vi "plot_init.vi"(10 "簇":T1, 11 "配置输入":T2 {"串口通信UI"."Format" items=["标准帧", "扩展帧"]; "串口通信UI"."Type" items=["数据帧", "远程帧"]; "串口通信UI"."ID" format="0x%x"; "串口通信UI"."Fliter" items=["接收所有类型"=1, "只接收标准帧"=2, "只接收扩展帧"=3]; "串口通信UI"."kBaudRate" items=["5k bps"=1, "10k bps"=2, "20k bps"=3, "40k bps"=4, "50k bps"=5, "80k bps"=6, "100k bps"=7, "125k bps"=8, "200k bps"=9, "250k bps"=10, "400k bps"=11, "500k bps"=12, "666k bps"=13, "800k bps"=14, "1000k bps"=15, "33.33k bps"=16, "66.66k bps"=17, "83.33k bps"=18]; "串口通信UI"."Mode" items=["正常工作", "仅侦听模式", "自测模式（环回）"]; "串口通信UI"."InitFlag" items=["使用界面设置参数"=1]; "串口通信UI"."AccMask" format="%08x"; "串口通信UI"."AccCode" format="%08x"; "串口通信UI"."Channel" items=["通道1", "通道2"]; "串口通信UI"."DevType" items=["USB-CAN"=3, "USB-CAN2"=4]; "安全报警UI"."操作 8" items=["产生报警信息（不发声），等待手动操作", "产生报警信息（发声），等待手动操作", "产生报警信息（不发声），自动刹车", "产生报警信息（发声），自动刹车", "产生报警信息（不发声），立即自动断电，开启泄放电阻", "产生报警信息（发声），立即自动断电，开启泄放电阻"]; "安全报警UI"."操作 7" items=["产生报警信息（不发声），等待手动操作", "产生报警信息（发声），等待手动操作", "产生报警信息（不发声），自动刹车", "产生报警信息（发声），自动刹车", "产生报警信息（不发声），立即自动断电，开启泄放电阻", "产生报警信息（发声），立即自动断电，开启泄放电阻"]; "安全报警UI"."操作 6" items=["产生报警信息（不发声），等待手动操作", "产生报警信息（发声），等待手动操作", "产生报警信息（不发声），自动刹车", "产生报警信息（发声），自动刹车", "产生报警信息（不发声），立即自动断电，开启泄放电阻", "产生报警信息（发声），立即自动断电，开启泄放电阻"]; "安全报警UI"."操作 5" items=["产生报警信息（不发声），等待手动操作", "产生报警信息（发声），等待手动操作", "产生报警信息（不发声），自动刹车", "产生报警信息（发声），自动刹车", "产生报警信息（不发声），立即自动断电，开启泄放电阻", "产生报警信息（发声），立即自动断电，开启泄放电阻"]; "安全报警UI"."操作 4" items=["产生报警信息（不发声），等待手动操作", "产生报警信息（发声），等待手动操作", "产生报警信息（不发声），自动刹车", "产生报警信息（发声），自动刹车", "产生报警信息（不发声），立即自动断电，开启泄放电阻", "产生报警信息（发声），立即自动断电，开启泄放电阻"]; "安全报警UI"."操作 3" items=["产生报警信息（不发声），等待手动操作", "产生报警信息（发声），等待手动操作", "产生报警信息（不发声），自动刹车", "产生报警信息（发声），自动刹车", "产生报警信息（不发声），立即自动断电，开启泄放电阻", "产生报警信息（发声），立即自动断电，开启泄放电阻"]; "安全报警UI"."操作 2" items=["产生报警信息（不发声），等待手动操作", "产生报警信息（发声），等待手动操作", "产生报警信息（不发声），自动刹车", "产生报警信息（发声），自动刹车", "产生报警信息（不发声），立即自动断电，开启泄放电阻", "产生报警信息（发声），立即自动断电，开启泄放电阻"]; "安全报警UI"."操作" items=["产生报警信息（不发声），等待手动操作", "产生报警信息（发声），等待手动操作", "产生报警信息（不发声），自动刹车", "产生报警信息（发声），自动刹车", "产生报警信息（不发声），立即自动断电，开启泄放电阻", "产生报警信息（发声），立即自动断电，开启泄放电阻"]}) -> (3 "配置输出":T2 {"串口通信UI"."Format" items=["标准帧", "扩展帧"]; "串口通信UI"."Type" items=["数据帧", "远程帧"]; "串口通信UI"."ID" format="0x%x"; "串口通信UI"."Fliter" items=["接收所有类型"=1, "只接收标准帧"=2, "只接收扩展帧"=3]; "串口通信UI"."kBaudRate" items=["5k bps"=1, "10k bps"=2, "20k bps"=3, "40k bps"=4, "50k bps"=5, "80k bps"=6, "100k bps"=7, "125k bps"=8, "200k bps"=9, "250k bps"=10, "400k bps"=11, "500k bps"=12, "666k bps"=13, "800k bps"=14, "1000k bps"=15, "33.33k bps"=16, "66.66k bps"=17, "83.33k bps"=18]; "串口通信UI"."Mode" items=["正常工作", "仅侦听模式", "自测模式（环回）"]; "串口通信UI"."InitFlag" items=["使用界面设置参数"=1]; "串口通信UI"."AccMask" format="%08x"; "串口通信UI"."AccCode" format="%08x"; "串口通信UI"."Channel" items=["通道1", "通道2"]; "串口通信UI"."DevType" items=["USB-CAN"=3, "USB-CAN2"=4]; "安全报警UI"."操作 8" items=["产生报警信息（不发声），等待手动操作", "产生报警信息（发声），等待手动操作", "产生报警信息（不发声），自动刹车", "产生报警信息（发声），自动刹车", "产生报警信息（不发声），立即自动断电，开启泄放电阻", "产生报警信息（发声），立即自动断电，开启泄放电阻"]; "安全报警UI"."操作 7" items=["产生报警信息（不发声），等待手动操作", "产生报警信息（发声），等待手动操作", "产生报警信息（不发声），自动刹车", "产生报警信息（发声），自动刹车", "产生报警信息（不发声），立即自动断电，开启泄放电阻", "产生报警信息（发声），立即自动断电，开启泄放电阻"]; "安全报警UI"."操作 6" items=["产生报警信息（不发声），等待手动操作", "产生报警信息（发声），等待手动操作", "产生报警信息（不发声），自动刹车", "产生报警信息（发声），自动刹车", "产生报警信息（不发声），立即自动断电，开启泄放电阻", "产生报警信息（发声），立即自动断电，开启泄放电阻"]; "安全报警UI"."操作 5" items=["产生报警信息（不发声），等待手动操作", "产生报警信息（发声），等待手动操作", "产生报警信息（不发声），自动刹车", "产生报警信息（发声），自动刹车", "产生报警信息（不发声），立即自动断电，开启泄放电阻", "产生报警信息（发声），立即自动断电，开启泄放电阻"]; "安全报警UI"."操作 4" items=["产生报警信息（不发声），等待手动操作", "产生报警信息（发声），等待手动操作", "产生报警信息（不发声），自动刹车", "产生报警信息（发声），自动刹车", "产生报警信息（不发声），立即自动断电，开启泄放电阻", "产生报警信息（发声），立即自动断电，开启泄放电阻"]; "安全报警UI"."操作 3" items=["产生报警信息（不发声），等待手动操作", "产生报警信息（发声），等待手动操作", "产生报警信息（不发声），自动刹车", "产生报警信息（发声），自动刹车", "产生报警信息（不发声），立即自动断电，开启泄放电阻", "产生报警信息（发声），立即自动断电，开启泄放电阻"]; "安全报警UI"."操作 2" items=["产生报警信息（不发声），等待手动操作", "产生报警信息（发声），等待手动操作", "产生报警信息（不发声），自动刹车", "产生报警信息（发声），自动刹车", "产生报警信息（不发声），立即自动断电，开启泄放电阻", "产生报警信息（发声），立即自动断电，开启泄放电阻"]; "安全报警UI"."操作" items=["产生报警信息（不发声），等待手动操作", "产生报警信息（发声），等待手动操作", "产生报警信息（不发声），自动刹车", "产生报警信息（发声），自动刹车", "产生报警信息（不发声），立即自动断电，开启泄放电阻", "产生报警信息（发声），立即自动断电，开启泄放电阻"]})   [LabVIEW 2018, in "UI.lvlib"]
uses:
  UI.lvlib
  Settings/Settings.ctl
  Acquisition/Hardware Configuration.ctl
  Acquisition/Signal Type.ctl
  Acquisition/Acquisition.lvlib
  Settings/Settings.lvlib
panel:
  # "参数配置文件"
  # "输入数据文件"
  # "EHA电机"
  # "模拟电机"
  # "注：每次运行实验时销毁现有所有图像"
  # "参数配置文件"
  # "输入数据文件"
  # "EHA电机"
  # "模拟电机"
  # "注：每次运行实验时销毁现有所有图像"
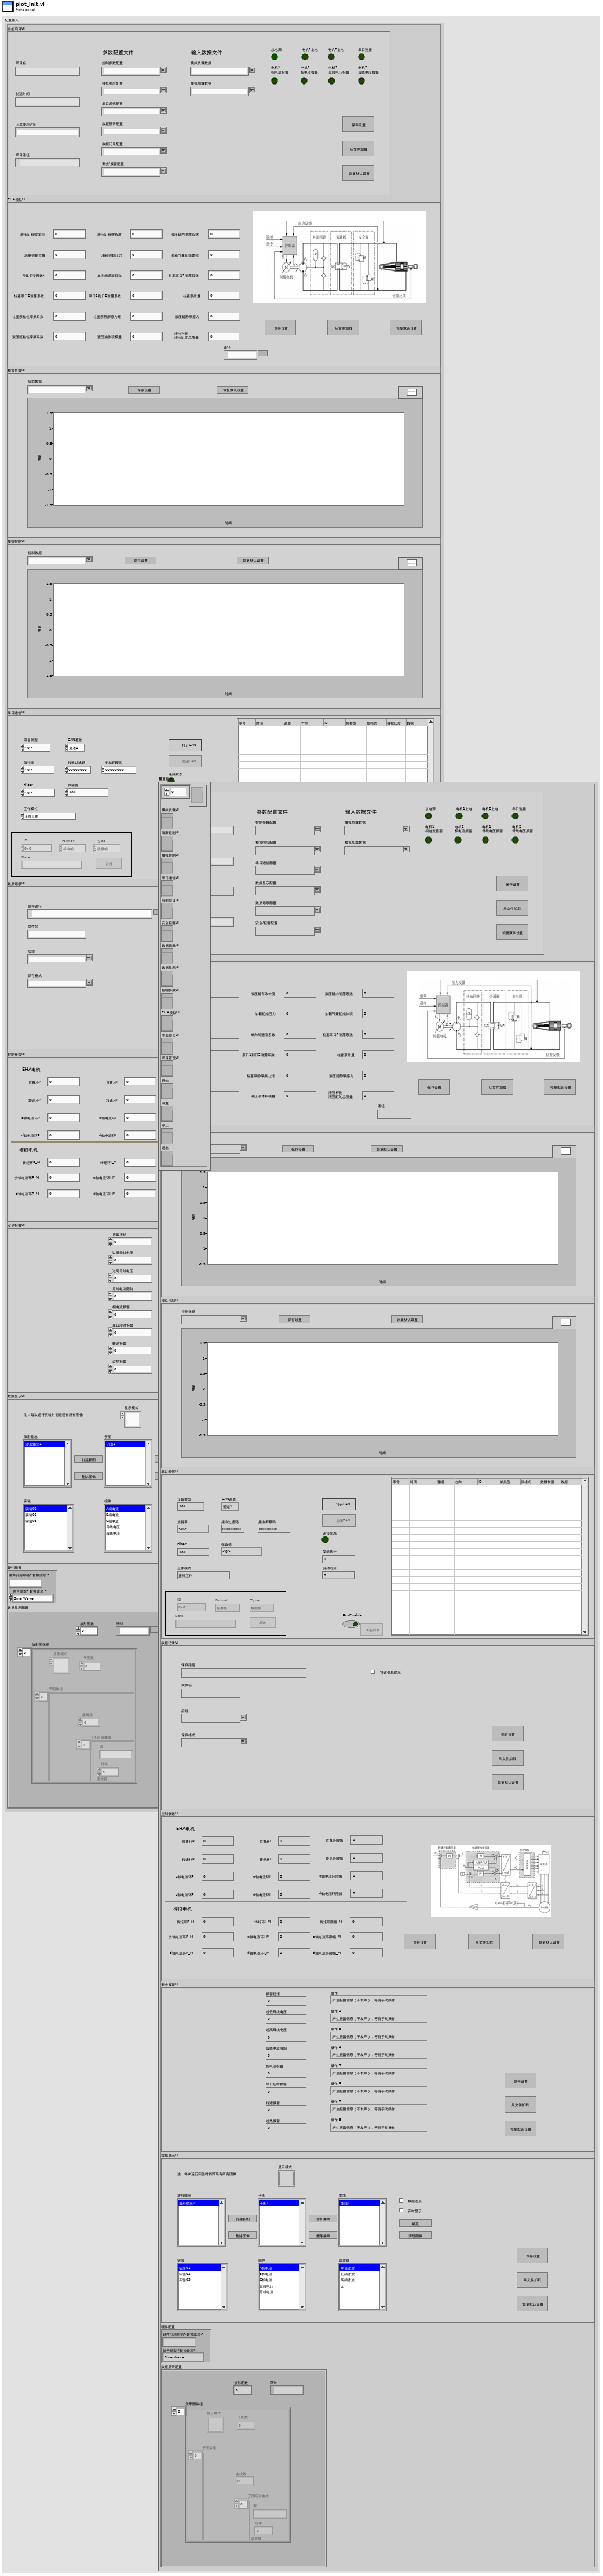
[diagram p1: front panel]
types:
  T1 = typedef "引用簇.ctl" = cluster{"数组":refnum<vi>[], "模拟负载UI":refnum<vi>, "波形控制UI":refnum<vi>, "模拟控制UI":refnum<vi>, "串口通信UI":refnum<vi>, "当前项目UI":refnum<vi>, "安全报警UI":refnum<vi>, "数据记录UI":refnum<vi>, "数据显示UI":refnum<vi>, "控制参数UI":refnum<vi>, "EHA模拟UI":refnum<vi>, "主选项卡UI":refnum<vi>, "项目管理UI":refnum<vi>, "开始":refnum<vi>, "设置":refnum<vi>, "停止":refnum<vi>, "退出":refnum<vi>}
  T2 = typedef "Settings.lvlib/Settings.ctl" = cluster{"当前项目UI":T3, "EHA模拟UI":T4, "模拟负载UI":T5, "模拟控制UI":T6, "串口通信UI":T7, "数据记录UI":T13, "控制参数UI":T14, "安全报警UI":T15, "数据显示UI":T16, "硬件配置":T17, "数据显示配置":T19}
  T3 = typedef "控件 5.ctl" = cluster{"控制参数配置":string, "模拟响应配置":string, "串口通信配置":string, "数据显示配置":string, "数据记录配置":string, "安全/报警配置":string, "模拟负载数据":string, "模拟加载数据":string, "总电源":bool, "电机1上电":bool, "电机2上电":bool, "串口连接":bool, "电机1\n相电流报警":bool, "电机2\n相电流报警":bool, "电机1\n母线电压报警":bool, "电机2\n母线电压报警":bool, "保存设置":bool, "从文件加载":bool, "恢复默认设置":bool, "路径":path, "项目路径":path, "项目名":string, "创建时间":string, "上次使用时间":string}
  T4 = typedef "EHA模拟UI.ctl" = cluster{"液压缸有效面积":dbl, "活塞初始位置":dbl, "气体多变系数k":dbl, "柱塞泵口2泄露系数":dbl, "柱塞泵粘性摩擦系数":dbl, "液压缸粘性摩擦系数":dbl, "液压缸有效长度":dbl, "油箱初始压力":dbl, "单向阀通流系数":dbl, "泵口1到口2泄露系数":dbl, "柱塞泵静摩擦力矩":dbl, "液压油体积模量":dbl, "保存设置":bool, "从文件加载":bool, "恢复默认设置":bool, "路径":path, "液压缸内泄露系数":dbl, "油箱气囊初始体积":dbl, "柱塞泵口1泄露系数":dbl, "柱塞泵排量":dbl, "液压缸静摩擦力":dbl, "液压杆到\n液压缸的总质量":dbl}
  T5 = typedef "控件 9.ctl" = cluster{"负载数据":string, "负载数据 2":waveform(dbl)[], "保存设置":bool, "恢复默认设置":bool}
  T6 = typedef "控件 7.ctl" = cluster{"控制数据":string, "负载数据 2":waveform(dbl)[], "保存设置":bool, "恢复默认设置":bool}
  T7 = typedef "控件 6.ctl" = cluster{"DevType":T8, "Channel":T9, "AccCode":u32, "AccMask":u32, "InitFlag":T10, "Mode":T11, "kBaudRate":u8, "Fliter":T12, "Open":bool, "Close":bool, "连接状态":bool, "SendCnt":u32, "RecvCnt":u32, "Send":bool, "ID":u32, "Data":string, "Type":u8, "Format":u8, "Clear":bool, "list":i32, "路径":path, "RcvEnable":bool}
  T8 = typedef "can库.lvlib/ControlCAN.lvlib/DevType.ctl" = u32
  T9 = typedef "can库.lvlib/ControlCAN.lvlib/CAN Channel.ctl" = u32
  T10 = typedef "can库.lvlib/ControlCAN.lvlib/InitFlag.ctl" = u32
  T11 = typedef "can库.lvlib/ControlCAN.lvlib/Mode.ctl" = u8
  T12 = typedef "can库.lvlib/ControlCAN.lvlib/Fliter.ctl" = u8
  T13 = typedef "控件 3.ctl" = cluster{"保存路径":path, "文件名":string, "后缀":string, "保存格式":string, "复选框":bool, "保存设置":bool, "从文件加载":bool, "恢复默认设置":bool, "路径":path, "TDMS文件引用":refnum<k34>}
  T14 = typedef "控件 1.ctl" = cluster{"d轴电流环P_M":dbl, "转速环P":dbl, "q轴电流环P":dbl, "d轴电流环P":dbl, "转矩环P_M":dbl, "去轴电流环P_M":dbl, "转速环I":dbl, "q轴电流环I":dbl, "d轴电流环I":dbl, "转矩环I_M":dbl, "q轴电流环I_M":dbl, "d轴电流环I_M":dbl, "保存设置":bool, "从文件加载":bool, "恢复默认设置":bool, "路径":path, "位置环P":dbl, "位置环I":dbl, "转速环限幅":dbl, "q轴电流环限幅":dbl, "d轴电流环限幅":dbl, "位置环限幅":dbl, "转矩环限幅_M":dbl, "q轴电流环限幅_M":dbl, "d轴电流环限幅_M":dbl}
  T15 = typedef "控件 4.ctl" = cluster{"报警扭矩":dbl, "过低母线电压":dbl, "过高母线电压":dbl, "母线电流限制":dbl, "相电流报警":dbl, "串口超时报警":dbl, "转速报警":dbl, "过热报警":dbl, "操作":u16, "操作 2":u16, "操作 3":u16, "操作 4":u16, "操作 5":u16, "操作 6":u16, "操作 7":u16, "操作 8":u16, "保存设置":bool, "从文件加载":bool, "恢复默认设置":bool, "路径":path}
  T16 = typedef "控件 2.ctl" = cluster{"保存设置":bool, "从文件加载":bool, "恢复默认设置":bool, "实验":i32, "波形输出":i32, "组件":i32, "曲线":i32, "滤波器":i32, "删除曲线":bool, "清理图像":bool, "添加曲线":bool, "数据选点":bool, "确定按钮":bool, "实时显示":bool, "子图":i32, "显示模式":u16, "路径":path, "删除图像":bool, "创建新图":bool}
  T17 = typedef "Acquisition.lvlib/Hardware Configuration.ctl" = cluster{"硬件引用句柄<替换此项>":string, "信号类型<替换该项>":T18}
  T18 = typedef "Acquisition.lvlib/Signal Type.ctl" = enum16{"Sine Wave", "Square with Noise"}
  T19 = typedef "波形图簇.ctl" = cluster{"波形图数":u32, "波形图数组":T20[], "路径":path}
  T20 = typedef "波形图.ctl" = cluster{"显示模式":u16, "子图数":u32, "子图数组":T21[]}
  T21 = typedef "子图.ctl" = cluster{"子图所有曲线":T22[], "曲线数":u32}
  T22 = typedef "曲线簇.ctl" = cluster{"源":string, "组件":u32, "滤波器":u32}
  T23 = typedef "主选项卡枚举常量.ctl" = enum32{"开始页", "当前项目配置", "串口通信配置", "控制参数配置", "EHA模拟配置", "模拟控制配置", "模拟负载配置", "安全报警配置", "数据显示配置", "数据记录配置", "波形输出1", "波形输出2", "波形输出3", "波形输出4", "波形输出5", "波形输出6"}
  T24 = typedef "组件常量.ctl" = string[]
  T25 = enum32{"开始页", "当前项目配置", "串口通信配置", "控制参数配置", "模拟响应配置", "模拟控制配置", "模拟负载配置", "安全报警配置", "数据显示配置", "数据记录配置", "波形输出1", "波形输出2", "波形输出3", "波形输出4", "波形输出5", "波形输出6"}
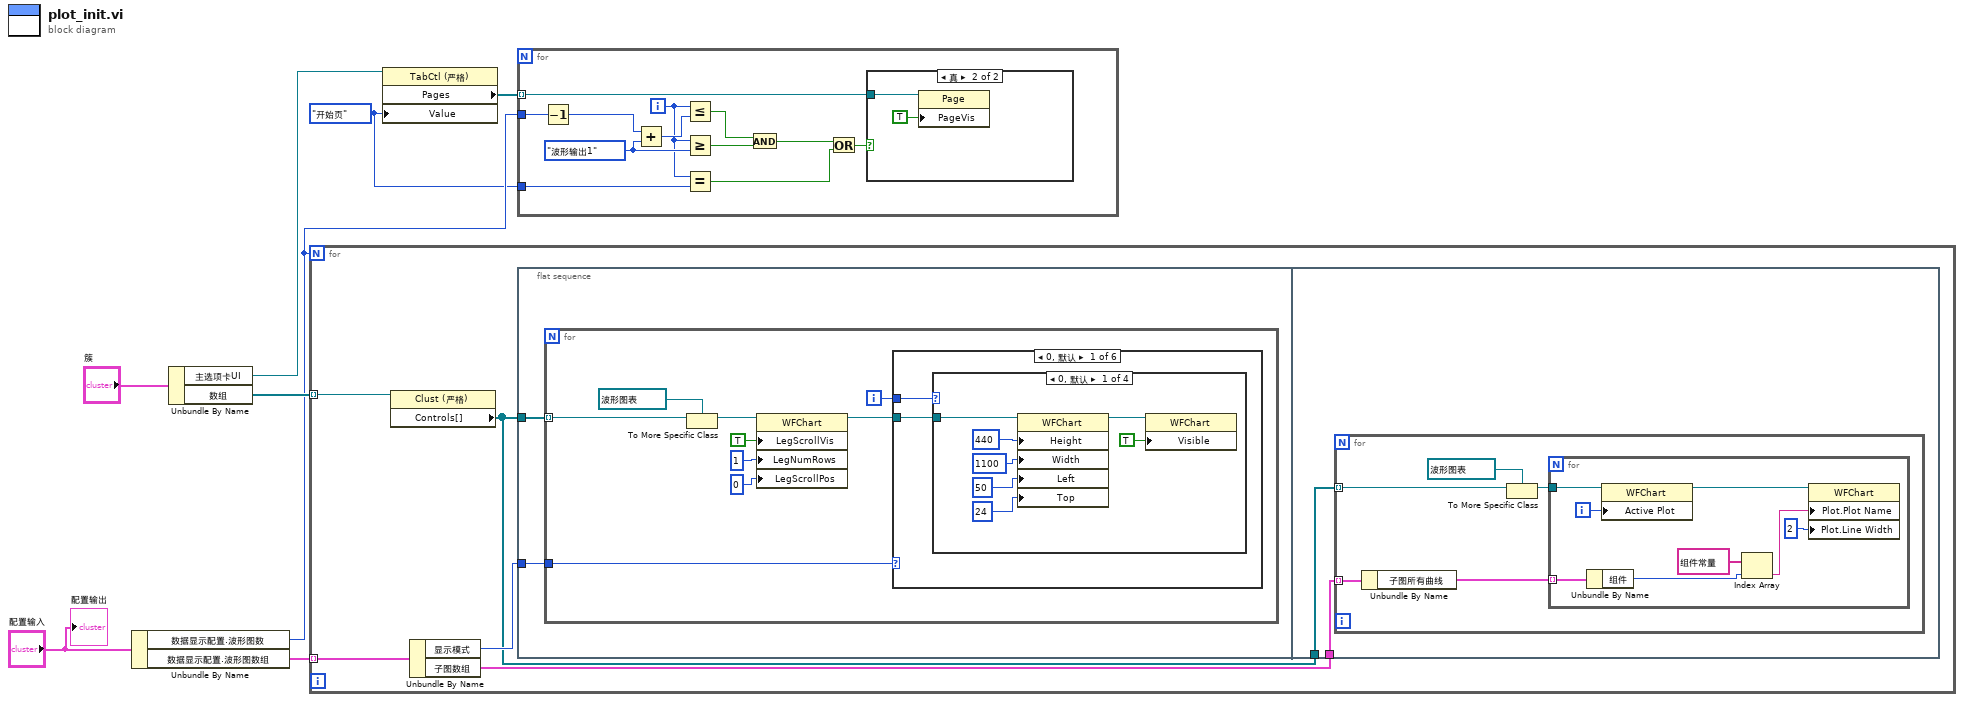
[diagram p0: block diagram]
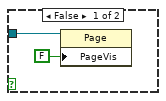
[diagram p2: hidden frame]
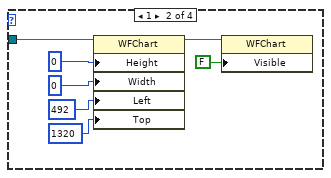
[diagram p3: hidden frame]
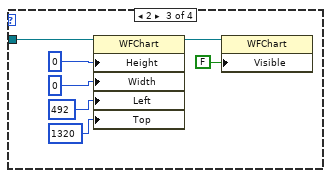
[diagram p4: hidden frame]
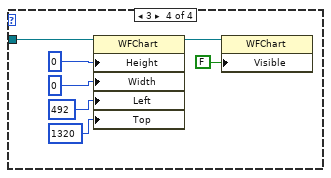
[diagram p5: hidden frame]
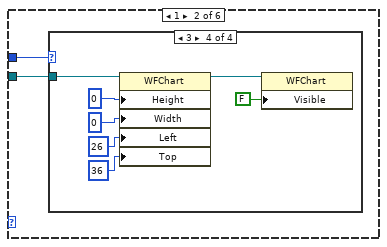
[diagram p6: hidden frame]
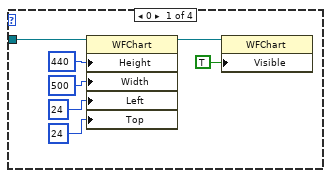
[diagram p7: hidden frame]
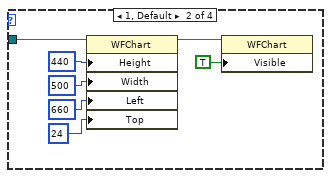
[diagram p8: hidden frame]
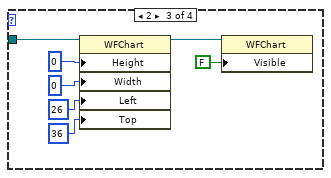
[diagram p9: hidden frame]
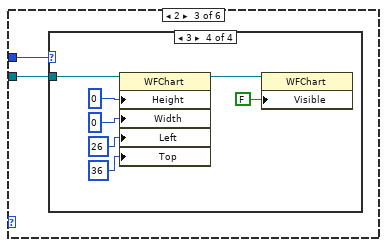
[diagram p10: hidden frame]
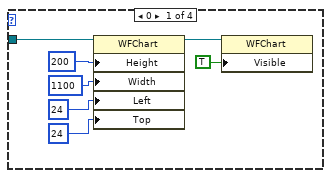
[diagram p11: hidden frame]
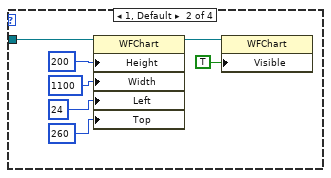
[diagram p12: hidden frame]
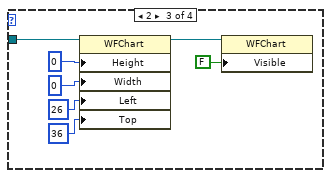
[diagram p13: hidden frame]
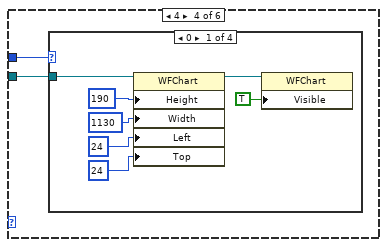
[diagram p14: hidden frame]
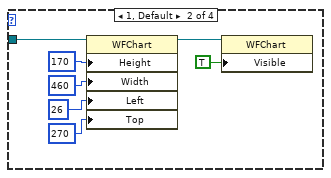
[diagram p15: hidden frame]
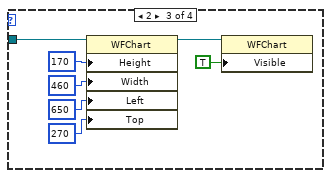
[diagram p16: hidden frame]
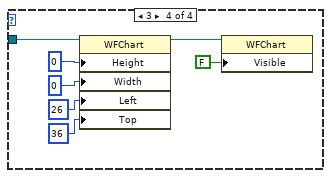
[diagram p17: hidden frame]
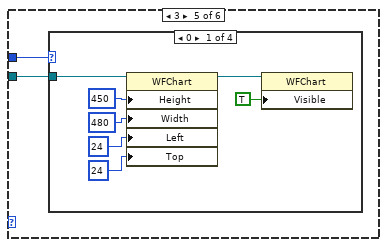
[diagram p18: hidden frame]
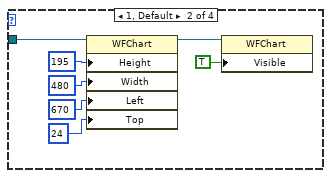
[diagram p19: hidden frame]
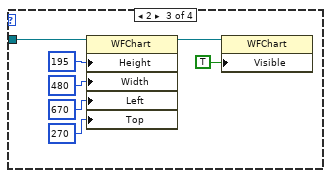
[diagram p20: hidden frame]
diagram:
  w1 = 主选项卡枚举常量."开始页" ("值")
  n1 = Unbundle By Name("配置输入") -> ("数据显示配置.波形图数"=w2:u32, "数据显示配置.波形图数组"=w6:T20[])
  n2 = Unbundle By Name("簇") -> ("主选项卡UI"=w4:refnum<vi>, "数组"=w5:refnum<vi>[])
  n3 = for {
    N: w2 -> [_]
    tunnel: w6 -> [w13] mode=indexing
    tunnel: w5 -> [w11] mode=indexing
    n4 = property class="Clust (严格)"(reference=w11) -> ("Controls[]"=w9:refnum<vi>[])  [unwired: 1 in, 2 out]
    n5 = Unbundle By Name(w13) -> ("显示模式"=w12:u16, "子图数组"=w10:T21[])
    n6 = flat-sequence {
      tunnel: w12 -> [w15]
      tunnel: w9 -> [w14]
      tunnel: w10 -> [w206]
      tunnel: w9 -> [w205]
      frame #0 {
        n7 = for {
          tunnel: w15 -> [w20]
          tunnel: w14 -> [w16] mode=indexing
          i -> [w19]
          n8 = To More Specific Class(target class=refnum<vi> refnum ("特定类引用"), reference=w16) -> (specific class reference=w18:refnum<vi>)  [unwired: 1 in, 1 out]
          n9 = property class="WFChart"(reference=w18, "LegScrollVis"=TRUE ("图例:滚动条可见"), "LegNumRows"=u32 1 ("图例:行数"), "LegScrollPos"=u32 0 ("图例:滚动条位置")) -> (reference out=w17:refnum<vi>)  [unwired: 1 in, 1 out]
          n10 = case shown="0, 默认" w20 {
            tunnel: w19 -> [w26 w56 w86 w116 w146 w176]
            tunnel: w17 -> [w25 w55 w85 w115 w145 w175]
            frame 0, Default {
              n11 = case shown="0, 默认" w26 {
                tunnel: w25 -> [w29 w34 w41 w48]
                frame 0, Default {
                  n12 = property class="WFChart"(reference=w29, "Height"=u32 440 ("绘图区域:大小:高度"), "Width"=u32 1100 ("绘图区域:大小:宽度"), "Left"=50 ("位置:居左"), "Top"=24 ("x")) -> (reference out=w27:refnum<vi>)  [unwired: 1 in, 1 out]
                  n13 = property class="WFChart"(reference=w27, "Visible"=TRUE ("可见")) -> ()  [unwired: 1 in, 2 out]
                }
                frame 1 {
                  n14 = property class="WFChart"(reference=w34, "Height"=u32 0 ("绘图区域:大小:高度"), "Width"=u32 0 ("绘图区域:大小:宽度"), "Left"=492 ("位置:居左"), "Top"=1320 ("x")) -> (reference out=w35:refnum<vi>)  [unwired: 1 in, 1 out]
                  n15 = property class="WFChart"(reference=w35, "Visible"=FALSE ("可见")) -> ()  [unwired: 1 in, 2 out]
                }
                frame 2 {
                  n16 = property class="WFChart"(reference=w41, "Height"=u32 0 ("绘图区域:大小:高度"), "Width"=u32 0 ("绘图区域:大小:宽度"), "Left"=492 ("位置:居左"), "Top"=1320 ("x")) -> (reference out=w42:refnum<vi>)  [unwired: 1 in, 1 out]
                  n17 = property class="WFChart"(reference=w42, "Visible"=FALSE ("可见")) -> ()  [unwired: 1 in, 2 out]
                }
                frame 3 {
                  n18 = property class="WFChart"(reference=w48, "Height"=u32 0 ("绘图区域:大小:高度"), "Width"=u32 0 ("绘图区域:大小:宽度"), "Left"=492 ("位置:居左"), "Top"=1320 ("x")) -> (reference out=w49:refnum<vi>)  [unwired: 1 in, 1 out]
                  n19 = property class="WFChart"(reference=w49, "Visible"=FALSE ("可见")) -> ()  [unwired: 1 in, 2 out]
                }
              }
            }
            frame 1 {
              n20 = case shown="3" w56 {
                tunnel: w55 -> [w57 w64 w71 w78]
                frame 0 {
                  n21 = property class="WFChart"(reference=w57, "Height"=u32 440 ("绘图区域:大小:高度"), "Width"=u32 500 ("绘图区域:大小:宽度"), "Left"=24 ("位置:居左"), "Top"=24 ("x")) -> (reference out=w58:refnum<vi>)  [unwired: 1 in, 1 out]
                  n22 = property class="WFChart"(reference=w58, "Visible"=TRUE ("可见")) -> ()  [unwired: 1 in, 2 out]
                }
                frame 1, Default {
                  n23 = property class="WFChart"(reference=w64, "Height"=u32 440 ("绘图区域:大小:高度"), "Width"=u32 500 ("绘图区域:大小:宽度"), "Left"=660 ("位置:居左"), "Top"=24 ("x")) -> (reference out=w65:refnum<vi>)  [unwired: 1 in, 1 out]
                  n24 = property class="WFChart"(reference=w65, "Visible"=TRUE ("可见")) -> ()  [unwired: 1 in, 2 out]
                }
                frame 2 {
                  n25 = property class="WFChart"(reference=w71, "Height"=u32 0 ("绘图区域:大小:高度"), "Width"=u32 0 ("绘图区域:大小:宽度"), "Left"=26 ("位置:居左"), "Top"=36 ("x")) -> (reference out=w72:refnum<vi>)  [unwired: 1 in, 1 out]
                  n26 = property class="WFChart"(reference=w72, "Visible"=FALSE ("可见")) -> ()  [unwired: 1 in, 2 out]
                }
                frame 3 {
                  n27 = property class="WFChart"(reference=w78, "Height"=u32 0 ("绘图区域:大小:高度"), "Width"=u32 0 ("绘图区域:大小:宽度"), "Left"=26 ("位置:居左"), "Top"=36 ("x")) -> (reference out=w79:refnum<vi>)  [unwired: 1 in, 1 out]
                  n28 = property class="WFChart"(reference=w79, "Visible"=FALSE ("可见")) -> ()  [unwired: 1 in, 2 out]
                }
              }
            }
            frame 2 {
              n29 = case shown="3" w86 {
                tunnel: w85 -> [w87 w94 w101 w108]
                frame 0 {
                  n30 = property class="WFChart"(reference=w87, "Height"=u32 200 ("绘图区域:大小:高度"), "Width"=u32 1100 ("绘图区域:大小:宽度"), "Left"=24 ("位置:居左"), "Top"=24 ("x")) -> (reference out=w88:refnum<vi>)  [unwired: 1 in, 1 out]
                  n31 = property class="WFChart"(reference=w88, "Visible"=TRUE ("可见")) -> ()  [unwired: 1 in, 2 out]
                }
                frame 1, Default {
                  n32 = property class="WFChart"(reference=w94, "Height"=u32 200 ("绘图区域:大小:高度"), "Width"=u32 1100 ("绘图区域:大小:宽度"), "Left"=24 ("位置:居左"), "Top"=260 ("x")) -> (reference out=w95:refnum<vi>)  [unwired: 1 in, 1 out]
                  n33 = property class="WFChart"(reference=w95, "Visible"=TRUE ("可见")) -> ()  [unwired: 1 in, 2 out]
                }
                frame 2 {
                  n34 = property class="WFChart"(reference=w101, "Height"=u32 0 ("绘图区域:大小:高度"), "Width"=u32 0 ("绘图区域:大小:宽度"), "Left"=26 ("位置:居左"), "Top"=36 ("x")) -> (reference out=w102:refnum<vi>)  [unwired: 1 in, 1 out]
                  n35 = property class="WFChart"(reference=w102, "Visible"=FALSE ("可见")) -> ()  [unwired: 1 in, 2 out]
                }
                frame 3 {
                  n36 = property class="WFChart"(reference=w108, "Height"=u32 0 ("绘图区域:大小:高度"), "Width"=u32 0 ("绘图区域:大小:宽度"), "Left"=26 ("位置:居左"), "Top"=36 ("x")) -> (reference out=w109:refnum<vi>)  [unwired: 1 in, 1 out]
                  n37 = property class="WFChart"(reference=w109, "Visible"=FALSE ("可见")) -> ()  [unwired: 1 in, 2 out]
                }
              }
            }
            frame 4 {
              n38 = case shown="0" w116 {
                tunnel: w115 -> [w117 w124 w131 w138]
                frame 0 {
                  n39 = property class="WFChart"(reference=w117, "Height"=u32 190 ("绘图区域:大小:高度"), "Width"=u32 1130 ("绘图区域:大小:宽度"), "Left"=24 ("位置:居左"), "Top"=24 ("x")) -> (reference out=w118:refnum<vi>)  [unwired: 1 in, 1 out]
                  n40 = property class="WFChart"(reference=w118, "Visible"=TRUE ("可见")) -> ()  [unwired: 1 in, 2 out]
                }
                frame 1, Default {
                  n41 = property class="WFChart"(reference=w124, "Height"=u32 170 ("绘图区域:大小:高度"), "Width"=u32 460 ("绘图区域:大小:宽度"), "Left"=26 ("位置:居左"), "Top"=270 ("x")) -> (reference out=w125:refnum<vi>)  [unwired: 1 in, 1 out]
                  n42 = property class="WFChart"(reference=w125, "Visible"=TRUE ("可见")) -> ()  [unwired: 1 in, 2 out]
                }
                frame 2 {
                  n43 = property class="WFChart"(reference=w131, "Height"=u32 170 ("绘图区域:大小:高度"), "Width"=u32 460 ("绘图区域:大小:宽度"), "Left"=650 ("位置:居左"), "Top"=270 ("x")) -> (reference out=w132:refnum<vi>)  [unwired: 1 in, 1 out]
                  n44 = property class="WFChart"(reference=w132, "Visible"=TRUE ("可见")) -> ()  [unwired: 1 in, 2 out]
                }
                frame 3 {
                  n45 = property class="WFChart"(reference=w138, "Height"=u32 0 ("绘图区域:大小:高度"), "Width"=u32 0 ("绘图区域:大小:宽度"), "Left"=26 ("位置:居左"), "Top"=36 ("x")) -> (reference out=w139:refnum<vi>)  [unwired: 1 in, 1 out]
                  n46 = property class="WFChart"(reference=w139, "Visible"=FALSE ("可见")) -> ()  [unwired: 1 in, 2 out]
                }
              }
            }
            frame 3 {
              n47 = case shown="0" w146 {
                tunnel: w145 -> [w147 w154 w161 w168]
                frame 0 {
                  n48 = property class="WFChart"(reference=w147, "Height"=u32 450 ("绘图区域:大小:高度"), "Width"=u32 480 ("绘图区域:大小:宽度"), "Left"=24 ("位置:居左"), "Top"=24 ("x")) -> (reference out=w148:refnum<vi>)  [unwired: 1 in, 1 out]
                  n49 = property class="WFChart"(reference=w148, "Visible"=TRUE ("可见")) -> ()  [unwired: 1 in, 2 out]
                }
                frame 1, Default {
                  n50 = property class="WFChart"(reference=w154, "Height"=u32 195 ("绘图区域:大小:高度"), "Width"=u32 480 ("绘图区域:大小:宽度"), "Left"=670 ("位置:居左"), "Top"=24 ("x")) -> (reference out=w155:refnum<vi>)  [unwired: 1 in, 1 out]
                  n51 = property class="WFChart"(reference=w155, "Visible"=TRUE ("可见")) -> ()  [unwired: 1 in, 2 out]
                }
                frame 2 {
                  n52 = property class="WFChart"(reference=w161, "Height"=u32 195 ("绘图区域:大小:高度"), "Width"=u32 480 ("绘图区域:大小:宽度"), "Left"=670 ("位置:居左"), "Top"=270 ("x")) -> (reference out=w162:refnum<vi>)  [unwired: 1 in, 1 out]
                  n53 = property class="WFChart"(reference=w162, "Visible"=TRUE ("可见")) -> ()  [unwired: 1 in, 2 out]
                }
                frame 3 {
                  n54 = property class="WFChart"(reference=w168, "Height"=u32 0 ("绘图区域:大小:高度"), "Width"=u32 0 ("绘图区域:大小:宽度"), "Left"=26 ("位置:居左"), "Top"=36 ("x")) -> (reference out=w169:refnum<vi>)  [unwired: 1 in, 1 out]
                  n55 = property class="WFChart"(reference=w169, "Visible"=FALSE ("可见")) -> ()  [unwired: 1 in, 2 out]
                }
              }
            }
            frame 5 {
              n56 = case shown="3" w176 {
                tunnel: w175 -> [w177 w184 w191 w198]
                frame 0 {
                  n57 = property class="WFChart"(reference=w177, "Height"=u32 180 ("绘图区域:大小:高度"), "Width"=u32 480 ("绘图区域:大小:宽度"), "Left"=26 ("位置:居左"), "Top"=30 ("x")) -> (reference out=w178:refnum<vi>)  [unwired: 1 in, 1 out]
                  n58 = property class="WFChart"(reference=w178, "Visible"=TRUE ("可见")) -> ()  [unwired: 1 in, 2 out]
                }
                frame 1, Default {
                  n59 = property class="WFChart"(reference=w184, "Height"=u32 180 ("绘图区域:大小:高度"), "Width"=u32 480 ("绘图区域:大小:宽度"), "Left"=670 ("位置:居左"), "Top"=30 ("x")) -> (reference out=w185:refnum<vi>)  [unwired: 1 in, 1 out]
                  n60 = property class="WFChart"(reference=w185, "Visible"=TRUE ("可见")) -> ()  [unwired: 1 in, 2 out]
                }
                frame 2 {
                  n61 = property class="WFChart"(reference=w191, "Height"=u32 180 ("绘图区域:大小:高度"), "Width"=u32 480 ("绘图区域:大小:宽度"), "Left"=26 ("位置:居左"), "Top"=270 ("x")) -> (reference out=w193:refnum<vi>)  [unwired: 1 in, 1 out]
                  n62 = property class="WFChart"(reference=w193, "Visible"=TRUE ("可见")) -> ()  [unwired: 1 in, 2 out]
                }
                frame 3 {
                  n63 = property class="WFChart"(reference=w198, "Height"=u32 180 ("绘图区域:大小:高度"), "Width"=u32 480 ("绘图区域:大小:宽度"), "Left"=670 ("位置:居左"), "Top"=270 ("x")) -> (reference out=w199:refnum<vi>)  [unwired: 1 in, 1 out]
                  n64 = property class="WFChart"(reference=w199, "Visible"=TRUE ("可见")) -> ()  [unwired: 1 in, 2 out]
                }
              }
            }
          }
        }
      }
      frame #1 {
        n65 = for {
          tunnel: w206 -> [w211] mode=indexing
          tunnel: w205 -> [w208] mode=indexing
          n66 = Unbundle By Name(w211) -> ("子图所有曲线"=w210:T22[])
          n67 = To More Specific Class(target class=refnum<vi> refnum ("特定类引用"), reference=w208) -> (specific class reference=w207:refnum<vi>)  [unwired: 1 in, 1 out]
          n68 = for {
            tunnel: w210 -> [w219] mode=indexing
            tunnel: w207 -> [w212]
            i -> [w218]
            n69 = Unbundle By Name(w219) -> ("组件"=w215:u32)
            n70 = property class="WFChart"(reference=w212, "Active Plot"=w218) -> (reference out=w217:refnum<vi>)  [unwired: 1 in, 1 out]
            n71 = Index Array(array=T24 ["正弦", "方波", "三角", "锯齿"] ("数组"), index=w215) -> (element=w214:string)
            n72 = property class="WFChart"(reference=w217, "Plot.Plot Name"=w214, "Plot.Line Width"=2) -> ()  [unwired: 1 in, 2 out]
          }
        }
      }
    }
  }
  n73 = property class="TabCtl (严格)"(reference=w4, "Value"=w1) -> ("Pages"=w3:refnum<vi>[])  [unwired: 1 in, 2 out]
  n74 = for {
    tunnel: w3 -> [w225] mode=indexing
    tunnel: w2 -> [w230]
    tunnel: w1 -> [w220]
    i -> [w222]
    w231 = T25."波形输出1" ("值")
    n75 = Decrement(x=w230) -> (x-1=w229:u32)
    n76 = Add(x=w229, y=w231) -> (x+y=w228:u32)
    n77 = Less Or Equal?(x=w222, y=w228) -> (x <= y?=w227:bool)
    n78 = Greater Or Equal?(x=w222, y=w231) -> (x >= y?=w226:bool)
    n79 = Equal?(x=w222, y=w220) -> (x = y?=w221:bool)
    n80 = And(x=w227, y=w226) -> (x .and. y?=w224:bool)
    n81 = Or(x=w224, y=w221) -> (x .or. y?=w223:bool)
    n82 = case shown="真" w223 {
      tunnel: w225 -> [w233 w235]
      frame False {
        n83 = property class="Page"(reference=w233, "PageVis"=FALSE ("选项卡可见")) -> ()  [unwired: 1 in, 2 out]
      }
      frame True {
        n84 = property class="Page"(reference=w235, "PageVis"=TRUE ("选项卡可见")) -> ()  [unwired: 1 in, 2 out]
      }
    }
  }
  "配置输出" <- "配置输入"
